vi "Process Connection.vi"(8 "error in (no error)":errorcluster, 10 "New Connection Policy":refnum<class "INewConnectionCallback.lvclass">, 11 "ConnectionFactoryHandler in":refnum<class "ConnectionFactoryHandler.lvclass">) -> (0 "error out":errorcluster, 3 "ConnectionFactoryHandler out":refnum<class "ConnectionFactoryHandler.lvclass">)   [LabVIEW 2019, in "ConnectionFactorySession.lvlib" / "ConnectionFactoryHandler.lvclass"]
uses:
  <vilib>/gpm_packages/@cs/Network-interface/Source/Connection Factory Session/ConnectionFactoryHandler/ConnectionFactoryHandler.lvclass
  C:/Program Files/National Instruments/LabVIEW 2019/vi.lib/gpm_packages/@cs/Network-interface/Source/Logged Actor/LoggedActor.lvclass
  C:/Program Files/National Instruments/LabVIEW 2019/vi.lib/ActorFramework/Actor/Actor.lvclass
  <vilib>/gpm_packages/@cs/Network-interface/Source/Connection Factory Session/INewConnectionCallback/INewConnectionCallback.lvclass
  <vilib>/gpm_packages/@cs/event-logger/Source/Composed Log/Types/Log Level.ctl
  <vilib>/gpm_packages/@cs/Network-interface/Source/Logged Actor/LoggedActor.lvclass/LoggedActor.ctl
  <vilib>/gpm_packages/@cs/event-logger/Source/Composed Log/LoggerReference/LoggerReference.lvclass/LoggerReference.ctl
  <vilib>/gpm_packages/@cs/Network-interface/Source/Connection Factory Session/ConnectionFactoryHandler/ConnectionFactoryHandler.lvclass/ConnectionFactoryHandler.ctl
  <vilib>/ActorFramework/Actor/Actor.lvclass/Actor.ctl
  <vilib>/ActorFramework/Message Enqueuer/Message Enqueuer.lvclass/Message Enqueuer.ctl
  <vilib>/gpm_packages/@cs/Network-interface/Source/Connection Factory Session/Messages/Create Connection Msg/Send Create Connection.vi
  <vilib>/ActorFramework/Actor/Read Self Enqueuer.vi
  <vilib>/gpm_packages/@cs/Network-interface/Source/Connection Factory Session/ConnectionFactoryHandler/Update Connection Cache.vi
  <vilib>/gpm_packages/@cs/event-logger/Source/Composed Log/LoggerReference/Log Event.vi
  <vilib>/ActorFramework/Message Enqueuer/Enqueue.vi
  <vilib>/ActorFramework/Message Enqueuer/Init from Existing Queue.vi
  <vilib>/gpm_packages/@cs/event-logger/Source/Composed Log/LoggerReference/Log.vi
  <vilib>/gpm_packages/@cs/event-logger/Source/Composed Log/LoggerReference/Get Valid Event Time.vi
  <vilib>/gpm_packages/@cs/event-logger/Source/Composed Log/LoggerReference/Remove Stale Logs.vi
  <vilib>/gpm_packages/@cs/Network-interface/Source/Connection Factory Session/Messages/Create Connection Msg/Create Connection Msg.lvclass
  C:/Program Files/National Instruments/LabVIEW 2019/vi.lib/ActorFramework/Message/Message.lvclass
  <vilib>/gpm_packages/@cs/Network-interface/Source/Connection Reference/Connection Reference/Construct Connection Reference.vi
  <vilib>/gpm_packages/@cs/Network-interface/Source/Connection Reference/Connection Reference/Close Connection.vi
  <vilib>/ActorFramework/Message Priority Queue/Priority Enqueue.vi
  <vilib>/gpm_packages/@cs/Network-interface/Source/Connection Reference/IConnection/IConnection.lvclass
  <vilib>/gpm_packages/@cs/Network-interface/Source/Connection Reference/Connection Reference/Connection Reference.lvclass
  <vilib>/ActorFramework/Message Enqueuer/Message Enqueuer.lvclass
  <vilib>/gpm_packages/@cs/Network-interface/Source/IConnectionFactory/IConnectionFactory.lvclass
  <vilib>/gpm_packages/@cs/Network-interface/Source/Logged Actor/LoggedActor.lvclass
  <vilib>/gpm_packages/@cs/event-logger/Source/Composed Log/Composed Log.lvlib
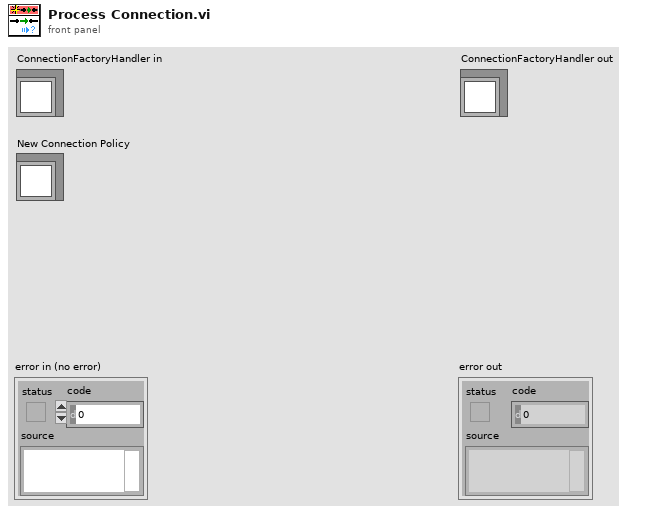
[diagram p1: front panel]
types:
  T1 = typedef "Composed Log.lvlib/Log Level.ctl" = enum16{"Debug", "Info", "Warning", "Error", "Critical"}
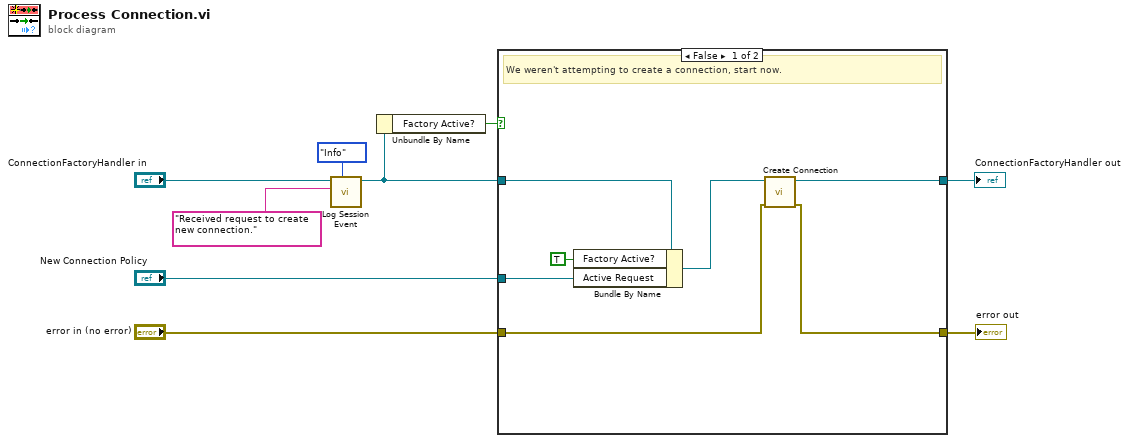
[diagram p0: block diagram]
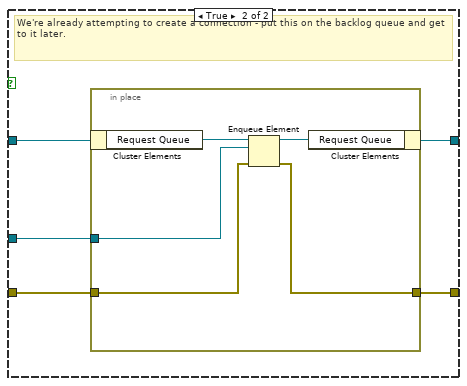
[diagram p2: hidden frame]
diagram:
  n1 = call <vilib>:"Log Session Event.vi"("Event Level"=Log_Level."Info", "Event Data"="Received request to create new connection.", "SessionActor in"="ConnectionFactoryHandler in") -> ("SessionActor out"=w3:refnum<class "ConnectionFactoryHandler.lvclass">)  [unwired: 7 in, 1 out]
  n2 = Unbundle By Name(w3) -> ("Factory Active?"=w9:bool)
  n3 = case shown="False" w9 {
    tunnel: "error in (no error)" -> [w12 w19]
    tunnel: w3 -> [w15 w21]
    tunnel: [w13 w17] -> w7
    tunnel: [w11 w18] -> w6
    tunnel: "New Connection Policy" -> [w16 w20]
    frame False {
      # "We weren't attempting to create a connection, start now."
      n4 = Bundle By Name(cluster=w15, "Factory Active?"=TRUE, "Active Request"=w16) -> (w14:refnum<class "ConnectionFactoryHandler.lvclass">)
      n5 = call <vilib>:"Create Connection.vi"("error in (no error)"=w12, "ConnectionFactoryHandler in"=w14) -> ("error out"=w11:errorcluster, "ConnectionFactoryHandler out"=w13:refnum<class "ConnectionFactoryHandler.lvclass">)  [unwired: 8 in]
    }
    frame True {
      # "We're already attempting to create a connection - put this on the backlog queue and get to it later."
      n6 = in-place {
        in-place-border: w20 -> [w24]
        in-place-border: w19 -> [w23]
        in-place-border: [w22] -> w18
        n7 = in-place-cluster #1(w21) -> ("Request Queue"=w26:refnum<queue>)
        n8 = Enqueue Element(queue=w26, element=w24, error in (no error)=w23) -> (queue out=w25:refnum<queue>, error out=w22:errorcluster)  [unwired: 1 in, 1 out]
        n9 = in-place-cluster #1("Request Queue"=w25) -> (w17:refnum<class "ConnectionFactoryHandler.lvclass">)
      }
    }
  }
  "error out" <- w6
  "ConnectionFactoryHandler out" <- w7
